vi "SMO.Example.SetPumpState.vi"(8 "error in (no error)":errorcluster, 10 "Pump State":bool=TRUE, 11 "SMO.Example":refnum<class "SMO.Example.lvclass">) -> (0 "error out":errorcluster, 3 "SMO.Example out":refnum<class "SMO.Example.lvclass">)   [LabVIEW 2013, in "SMO.Example.lvclass"]
doc: "---------------------------------------------------------------\nJKI State Machine Objects™\nhttp://jki.net/state-machine-objects/\nCopyright (C) 2005-2015, JKI <info@jki.net>\nALL RIGHTS RESERVED"
uses:
  SMO.Example.lvclass
  Typedefs/PumpState--Cluster.ctl
panel:
  # "For instructions on how to use the JKI State Machine Objects, examples and video tutorials, visit:\nhttp://jki.net/state-machine-objects/\n\nJKI State Machine Objects™\nhttp://jki.net/state-machine-objects/\nCopyright (C) 2005-2015, JKI <info@jki.net>\nALL RIGHTS RESERVED"
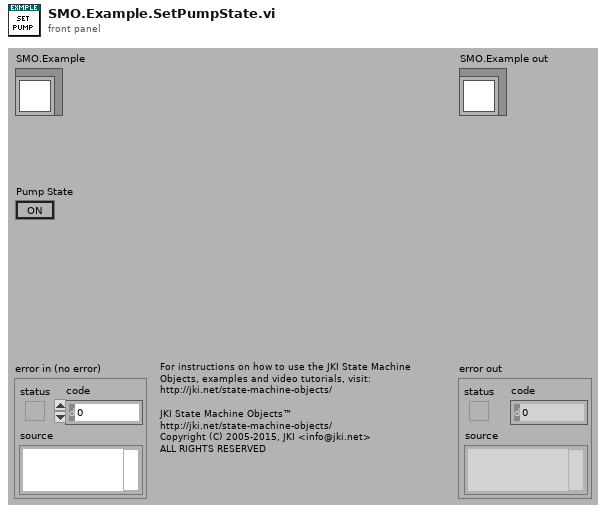
[diagram p1: front panel]
types:
  T1 = typedef "SMO.Example.lvclass/PumpState--Cluster.ctl" = cluster{"State":bool}
  T2 = typedef "SMO.Example.lvclass/ProtectedEvents--Cluster.ctl" = cluster{"API_Template":refnum<user-event>, "PumpState":refnum<user-event>, "Valve State":refnum<user-event>}
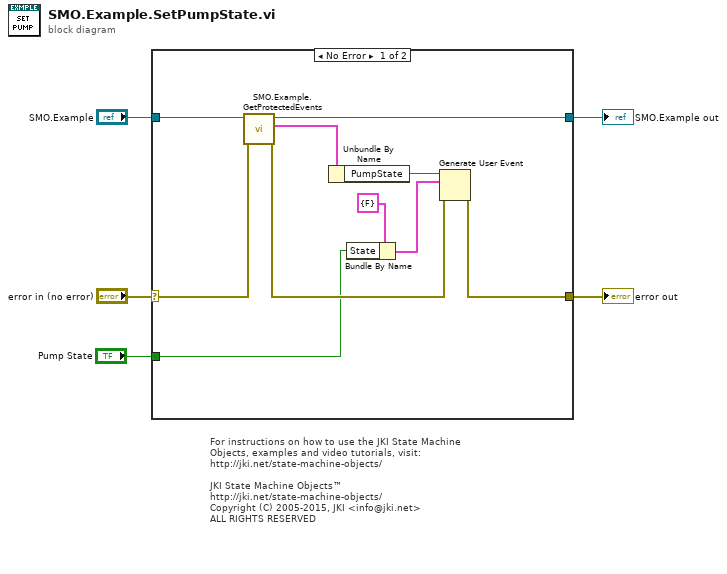
[diagram p0: block diagram]
diagram:
  # "For instructions on how to use the JKI State Machine Objects, examples and video tutorials, visit:\nhttp://jki.net/state-machine-objects/\n\nJKI State Machine Objects™\nhttp://jki.net/state-machine-objects/\nCopyright (C) 2005-2015, JKI <info@jki.net>\nALL RIGHTS RESERVED"
  n1 = case shown="No Error" "error in (no error)" {
    selector: "error in (no error)" -> [w13 w16]
    tunnel: "SMO.Example" -> [w15 w17]
    tunnel: [w9 w16] -> w4
    tunnel: [w14 w17] -> w3
    tunnel: "Pump State" -> [w7 _]
    frame No Error {
      n2 = call "SMO.Example.GetProtectedEvents.vi"("error in (no error)"=w13, "SMO.Example"=w15) -> ("error out"=w10:errorcluster, "Protected Events"=w12:T2, "SMO.Example out"=w14:refnum<class "SMO.Example.lvclass">)  [unwired: 7 in]
      n3 = Unbundle By Name(w12) -> ("PumpState"=w11:refnum<user-event>)
      n4 = Bundle By Name(cluster=T1 {"State"=FALSE} ("event data"), "State"=w7) -> (w6:T1)
      n5 = Generate User Event(user event=w11, event data cluster=w6, error in=w10) -> (error out=w9:errorcluster)  [unwired: 1 in, 1 out]
    }
    frame Error {
    }
  }
  "error out" <- w4
  "SMO.Example out" <- w3
